vi "Lookup Children by Meta Values.vi"(8 "error in (no error)":errorcluster, 9 "Meta Values":string[](array[string]), 10 "Meta Name":string, 11 "Config Element in":refnum<class "Config Element.lvclass">) -> (0 "error out":errorcluster, 1 "Names":string[](array[string]), 2 "Children":refnum<class "Config Element.lvclass">[](array[class]), 3 "Config Element out":refnum<class "Config Element.lvclass">)   [LabVIEW 2020, in "CDM-Config.lvlib" / "Config Element.lvclass"]
uses:
  Config Element.lvclass
  Config Element.lvclass/Config Element.ctl
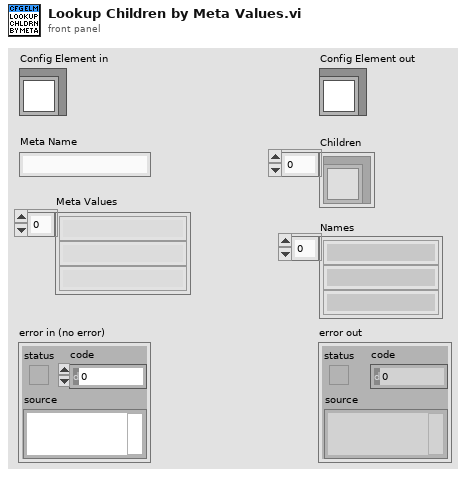
[diagram p1: front panel]
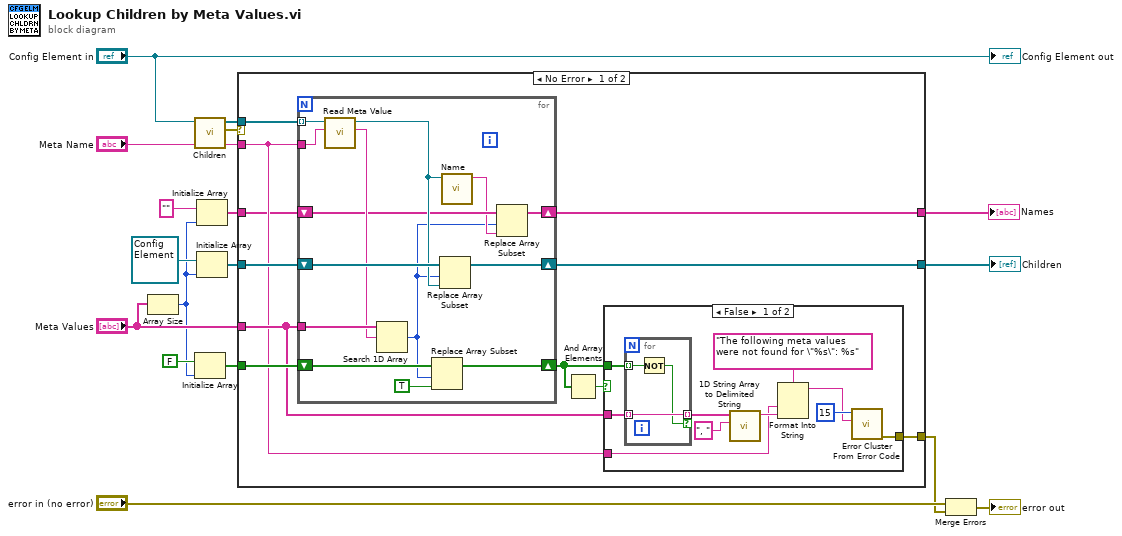
[diagram p0: block diagram]
diagram:
  n1 = Array Size(array="Meta Values") -> (size(s)=w4:i32)
  n2 = call "Children.vi"("Config Element in"="Config Element in") -> ("error out"=w7:errorcluster, "Elements"=w13:refnum<class "Config Element.lvclass">[])  [unwired: 9 in]
  n3 = Initialize Array(FALSE, w4) -> (w8:bool[])
  n4 = Initialize Array("", w4) -> (w2:string[])
  n5 = Initialize Array(refnum<class "Config Element.lvclass"> refnum ("Config Element in"), w4) -> (w14:refnum<class "Config Element.lvclass">[])
  n6 = case shown="No Error" w7 {
    selector: w7 -> [_ w56]
    tunnel: w14 -> [w28 _]
    tunnel: w13 -> [w27 _]
    tunnel: "Meta Values" -> [w22 _]
    tunnel: "Meta Name" -> [w21 _]
    tunnel: [w26 _] -> w10
    tunnel: w8 -> [w25 _]
    tunnel: [w20 w56] -> w5
    tunnel: w2 -> [w19 _]
    tunnel: [w18 _] -> w1
    frame No Error {
      n7 = for {
        shift-right: [w34] -> w26
        shift-left: w28 -> [w39]
        tunnel: w27 -> [w41] mode=indexing
        tunnel: w22 -> [w42]
        tunnel: w21 -> [w40]
        shift-right: [w35] -> w23
        shift-left: w25 -> [w37]
        shift-right: [w31] -> w18
        shift-left: w19 -> [w32]
        n8 = call "Read Meta Value.vi"("Meta Name"=w40, "Config Element in"=w41) -> ("Meta Value"=w38:string, "Config Element out"=w33:refnum<class "Config Element.lvclass">)  [unwired: 7 in, 1 out]
        n9 = Search 1D Array(1D array=w42, element=w38) -> (index of element=w29:i32)  [unwired: 1 in]
        n10 = Replace Array Subset(array=w37, new element=TRUE ("new element/subarray"), index=w29) -> (w35:bool[])
        n11 = Replace Array Subset(array=w39, new element=w33, index=w29) -> (w34:refnum<class "Config Element.lvclass">[])
        n12 = call "Name.vi"("Config Element in"=w33) -> ("Name"=w30:string)  [unwired: 9 in, 1 out]
        n13 = Replace Array Subset(array=w32, new element=w30, index=w29) -> (w31:string[])
      }
      n14 = And Array Elements(Boolean array=w23) -> (logical AND=w24:bool)
      n15 = case shown="False" w24 {
        tunnel: w23 -> [w52 _]
        tunnel: w22 -> [w51 _]
        tunnel: w21 -> [w47 _]
        tunnel: [w43 _] -> w20
        frame False {
          n16 = for {
            tunnel: w52 -> [w55] mode=indexing
            tunnel: w51 -> [w54] mode=indexing
            tunnel: [w54] -> w50 mode=indexing if=w53
            n17 = Not(x=w55) -> (.not. x?=w53:bool)
          }
          n18 = call <vilib>:"1D String Array to Delimited String.vi"("delimiter"=", ", "string array"=w50) -> ("delimited string"=w48:string)  [unwired: 9 in]
          n19 = Format Into String(format string="The following meta values were not found for \"%s\": %s", w47, w48) -> (resulting string=w44:string)  [unwired: 2 in, 1 out]
          n20 = call <vilib>:"Error Cluster From Error Code.vi"("error message (\"\")"=w44, "error code (0)"=15) -> ("error out"=w43:errorcluster)  [unwired: 7 in]
        }
        frame True {
          # "All values were found."
        }
      }
    }
    frame Error {
    }
  }
  "Children" <- w10
  "Names" <- w1
  n21 = Merge Errors("error in (no error)", w5) -> (→"error out":errorcluster)
  "Config Element out" <- "Config Element in"
